vi "SM1000-modulation.vi"(8 "error in (no error)":errorcluster, 11 "Object ref in":T1) -> (0 "error out":errorcluster, 3 "Object ref out":T1)   [LabVIEW 2013, in "HardwareCharacterization.lvlib" / "HC-Main.lvclass"]
uses:
  HC-Main.lvclass
  Object-reference.ctl
  HC-Main.lvclass/HC-Main.ctl
  Read SM1000.vi
  Read Scan file path.vi
  SM1000/HC-SM1000.lvclass
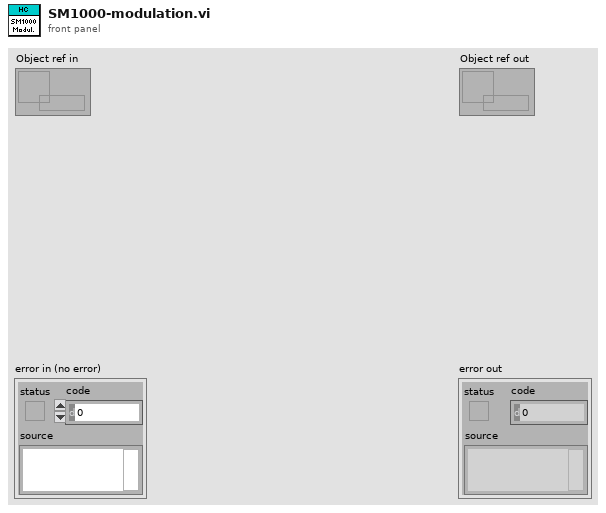
[diagram p1: front panel]
types:
  T1 = typedef "HardwareCharacterization.lvlib/HC-Main.lvclass/Object-reference.ctl" = refnum<data-value>
  T2 = typedef "HardwareCharacterization.lvlib/HC-SM1000.lvclass/Object-reference.ctl" = refnum<data-value>
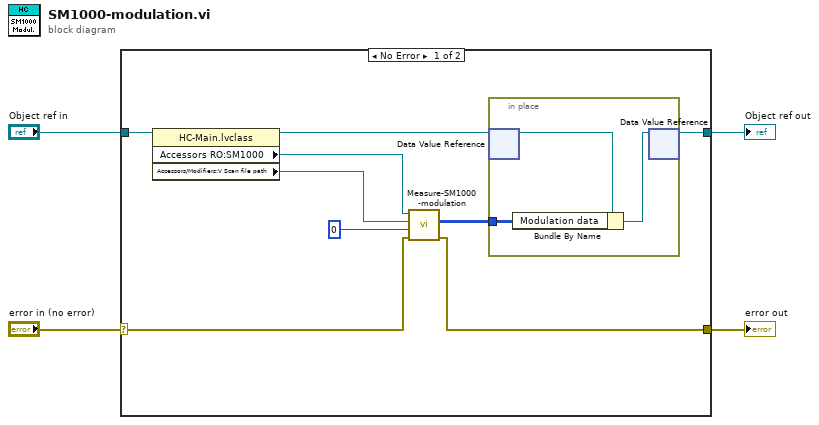
[diagram p0: block diagram]
diagram:
  n1 = case shown="No Error" "error in (no error)" {
    selector: "error in (no error)" -> [w9 w18]
    tunnel: [w8 w18] -> w3
    tunnel: [w5 w17] -> w1
    tunnel: "Object ref in" -> [w13 w17]
    frame No Error {
      n2 = property class="HC-Main.lvclass"(reference=w13) -> (reference out=w7:T1, "Accessors RO:SM1000"=w11:T2, "Accessors/Modifiers:V Scan file path"=w12:path)  [unwired: 1 in, 1 out]
      n3 = call "Measure-SM1000-modulation.vi"("error in (no error)"=w9, "Device index"=0, "File path"=w12, "SM1000-control in"=w11) -> ("error out"=w8:errorcluster, "Modulation data"=w6:i32[][])  [unwired: 5 in, 1 out]
      n4 = in-place {
        in-place-border: w6 -> [w16]
        n5 = in-place-dvr #1(w7) -> (w15:refnum<class "HC-Main.lvclass">)  [unwired: 1 out]
        n6 = Bundle By Name(cluster=w15, "Modulation data"=w16) -> (w14:refnum<class "HC-Main.lvclass">)
        n7 = in-place-dvr #1(w14) -> (w5:T1)  [unwired: 1 out]
      }
    }
    frame Error {
    }
  }
  "error out" <- w3
  "Object ref out" <- w1
